vi "Quad Encoder Out - FPGA.vi"(10 "Direction ?":bool, 11 "Period":u32) -> (2 "Period Count":u32, 3 "Current Period":u32)   [LabVIEW 8.6]
uses:
  <vilib>/eio/EIONode/EIONode.xnode
panel:
  in  "DIO 0":bool
  in  "DIO 1":bool
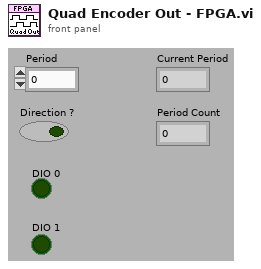
[diagram p1: front panel]
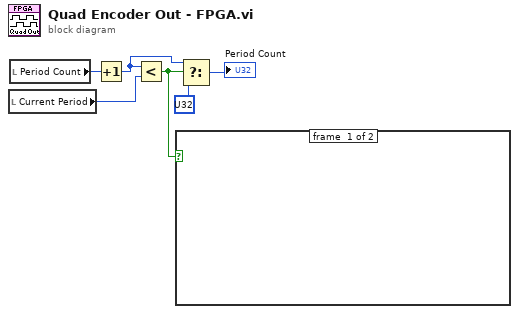
[diagram p0: block diagram]
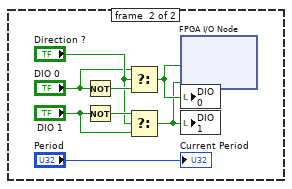
[diagram p2: hidden frame]
diagram:
  n1 = local read "Current Period"() -> (w6:u32)
  n2 = local read "Period Count"() -> (w3:u32)
  n3 = Increment(x=w3) -> (x+1=w4:u32)
  n4 = Less?(x=w4, y=w6) -> (x < y?=w2:bool)
  n5 = case shown="True" w2 {
    frame #0 {
    }
    frame #1 {
      n6 = Not(x="DIO 0") -> (.not. x?=w14:bool)
      n7 = Not(x="DIO 1") -> (.not. x?=w13:bool)
      n8 = Select(t="DIO 0", s="Direction ?", f=w14) -> (s? t:f=w11:bool)
      n9 = Select(t=w13, s="Direction ?", f="DIO 1") -> (s? t:f=w10:bool)
      n10 = xnode "FPGA I/O Node"("DIO0"=w11, "DIO1"=w10) -> ()  [unwired: 2 in, 2 out]
      n11 = local write "DIO 0"(w11) -> ()
      n12 = local write "DIO 1"(w10) -> ()
      "Current Period" <- "Period"
    }
  }
  n13 = Select(t=w4, s=w2, f=u32 ? ("t")) -> (s? t:f=→"Period Count":u32)
